vi "core_control_ref_from_name_error_handler.vi"(8 "error in":errorcluster, 9 "control names":string[](array[string]), 10 "found?":bool[](array[boolean]), 11 "vi ref":refnum<vi>) -> (0 "error out":errorcluster, 2 "found? duplicate":bool[](array[boolean]), 3 "vi ref dup":refnum<vi>)   [LabVIEW 2015, in "_ref_tools_polys.lvlib"]
uses:
  poly_ref_tools_eco_plus.vi
  _ref_tools_polys.lvlib
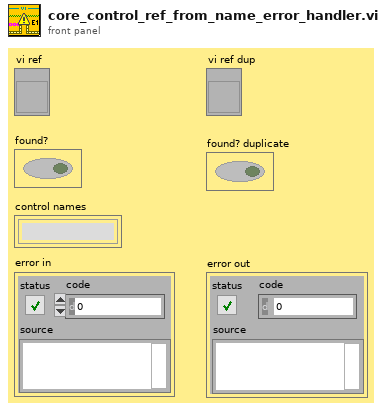
[diagram p1: front panel]
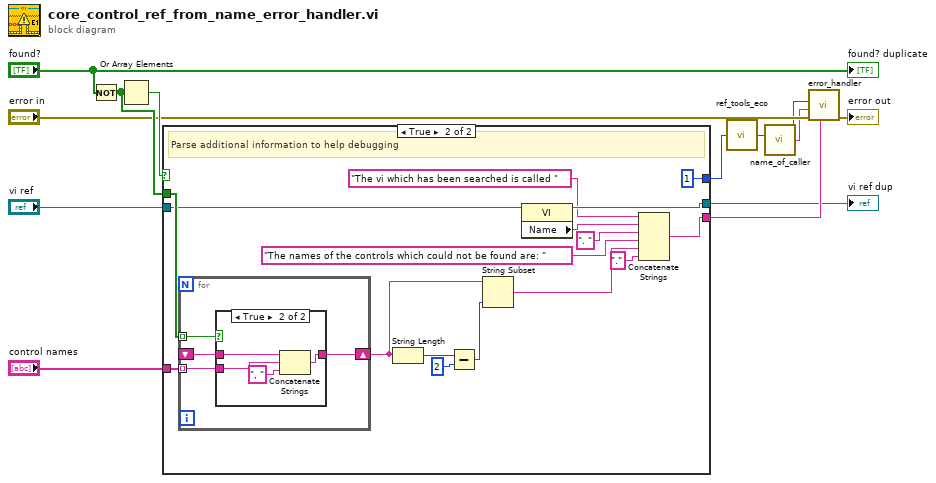
[diagram p0: block diagram]
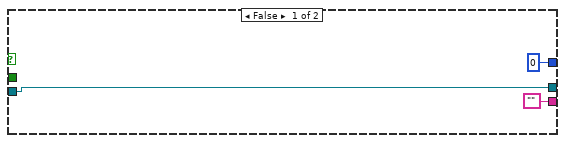
[diagram p2: hidden frame]
diagram:
  n1 = Not(x="found?") -> (.not. x?=w10:bool[])
  n2 = Or Array Elements(Boolean array=w10) -> (logical OR=w12:bool)
  n3 = case shown="True" w12 {
    tunnel: [0 1] -> w5
    tunnel: w10 -> [_ w30]
    tunnel: "control names" -> [_ w29]
    tunnel: ["" w22] -> w11
    tunnel: "vi ref" -> [w13 w21]
    tunnel: [w13 w20] -> w8
    frame False {
    }
    frame True {
      # "Parse additional information to help debugging"
      n4 = for {
        tunnel: w30 -> [w33] mode=indexing
        tunnel: w29 -> [w35] mode=indexing
        shift-right: [w34] -> w26
        shift-left: _ -> [w32]
        n5 = case shown="True" w33 {
          tunnel: w35 -> [_ w40]
          tunnel: [w36 w39] -> w34
          tunnel: w32 -> [w36 w38]
          frame False {
          }
          frame True {
            n6 = Concatenate Strings(w38, w40, ", " ("string")) -> (w39:string)
          }
        }
      }
      n7 = String Length(string=w26) -> (length=w25:i32)
      n8 = Subtract(x=w25, y=2) -> (x-y=w23:i32)
      n9 = String Subset(string=w26, length (rest)=w23) -> (substring=w27:string)  [unwired: 1 in]
      n10 = property class="VI"(reference=w21) -> (reference out=w20:refnum<vi>, "Name"=w18:string)  [unwired: 1 in, 1 out]
      n11 = Concatenate Strings("The vi which has been searched is called ", w18, ". " ("string"), "The names of the controls which could not be found are: ", w27, "." ("string")) -> (w22:string)
    }
  }
  "vi ref dup" <- w8
  n12 = call-poly "ref_tools_eco.vi"("code (w/out eco)"=w5) -> ("code (+ eco)"=w4:i32)  [unwired: 4 in]
  n13 = call "name_of_caller.vi"() -> ("name of caller out"=w3:string)  [unwired: 4 in]
  n14 = call "error_handler.vi"("Additional info"=w11, "error in (no error)"="error in", "name of caller in (you)"=w3, "code (0 = no error)"=w4) -> ("error out"=→"error out":errorcluster)  [unwired: 6 in, 1 out]
  "found? duplicate" <- "found?"
